vi "generateTiffStack.vi"() -> ()   [LabVIEW 2015]
panel:
  in  "Real":i32
  out "error out":errorcluster
  in  "error in":errorcluster
  in  "stackFnameArray":path[][][](array[path])
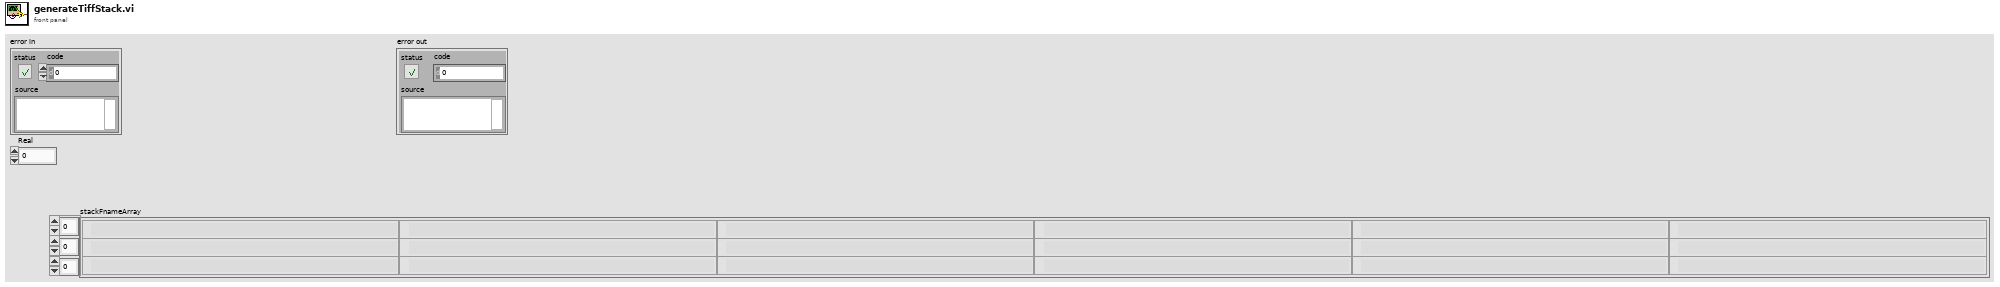
[diagram p1: front panel]
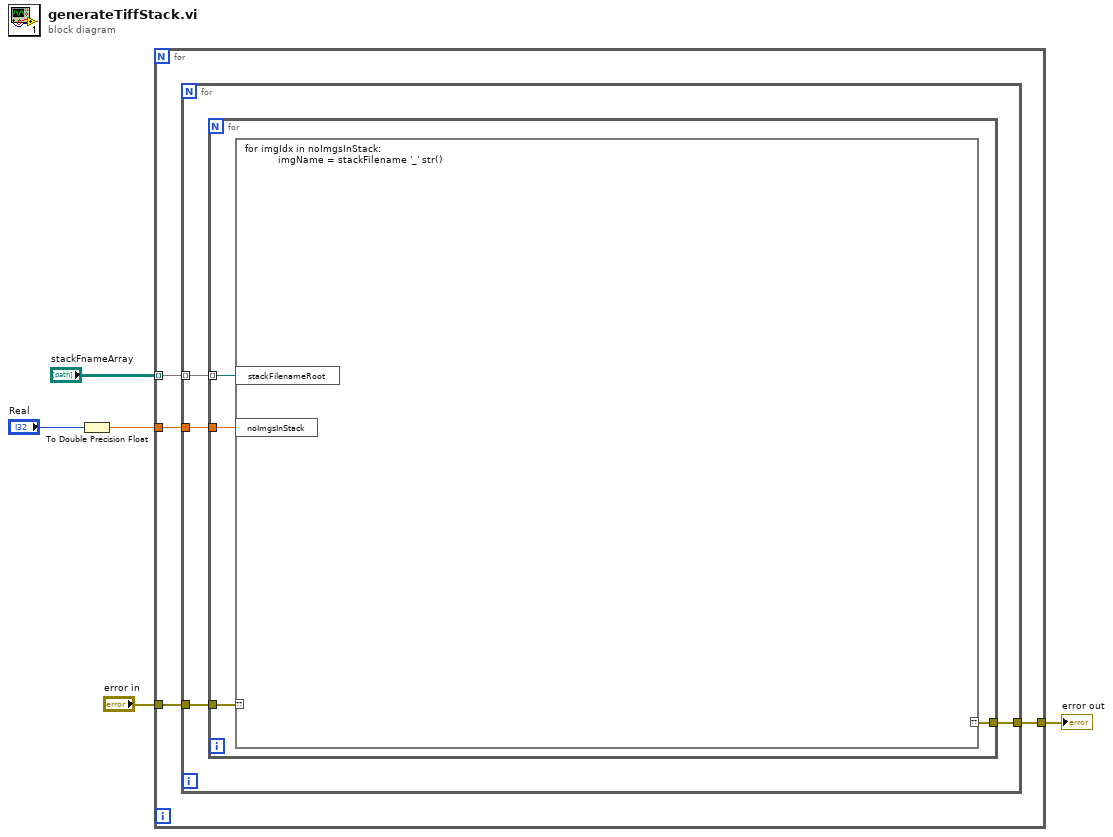
[diagram p0: block diagram]
diagram:
  n1 = To Double Precision Float(number="Real") -> (double precision float=w1:dbl)
  n2 = for {
    tunnel: "stackFnameArray" -> [w9] mode=indexing
    tunnel: "error in" -> [w8]
    tunnel: [w7] -> w3
    tunnel: w1 -> [w6]
    n3 = for {
      tunnel: w9 -> [w13] mode=indexing
      tunnel: w8 -> [w12]
      tunnel: [w11] -> w7
      tunnel: w6 -> [w10]
      n4 = for {
        tunnel: w13 -> [w17] mode=indexing
        tunnel: w12 -> [w16]
        tunnel: [w15] -> w11
        tunnel: w10 -> [w14]
        n5 = script code="for imgIdx in noImgsInStack:\n           imgName = stackFilename '_' str()"("??"=w16, "stackFilenameRoot"=w17, "noImgsInStack"=w14) -> ("??"=w15:errorcluster)
      }
    }
  }
  "error out" <- w3
